vi "Set Height.vi"(8 "Error In":errorcluster, 10 "Height":u32, 11 "Square In":refnum<class "Square.lvclass">) -> (0 "Error Out":errorcluster, 3 "Square Out":refnum<class "Square.lvclass">)   [LabVIEW 2019, in "Square.lvclass"]
uses:
  Square.lvclass
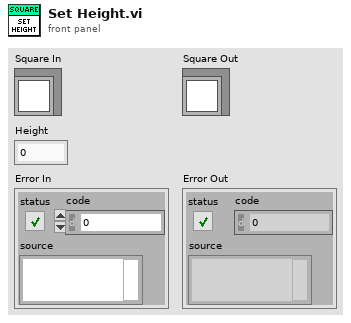
[diagram p1: front panel]
types:
  T1 = typedef "Square.lvclass/Data.ctl" = cluster{"Height":u32, "Width":u32}
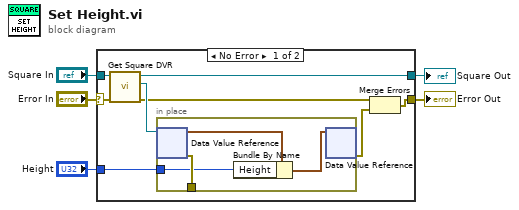
[diagram p0: block diagram]
diagram:
  n1 = case shown="No Error" "Error In" {
    selector: "Error In" -> [w9 w18]
    tunnel: [w12 w18] -> w4
    tunnel: [w7 w19] -> w2
    tunnel: "Square In" -> [w10 w19]
    tunnel: "Height" -> [w11 _]
    frame No Error {
      n2 = call "Get Square DVR.vi"("Error In"=w9, "Square In"=w10) -> ("Error Out"=w6:errorcluster, "DVR"=w8:refnum<data-value>, "Square Out"=w7:refnum<class "Square.lvclass">)  [unwired: 7 in]
      n3 = in-place {
        in-place-border: [w17] -> _
        in-place-border: w11 -> [w14]
        n4 = in-place-dvr #1(w8) -> (w16:T1, w17:errorcluster)
        n5 = Bundle By Name(cluster=w16, "Height"=w14) -> (w15:T1)
        n6 = in-place-dvr #1(w15) -> (w13:errorcluster)  [unwired: 1 out]
      }
      n7 = Merge Errors(w6, w13) -> (w12:errorcluster)
    }
    frame Error {
    }
  }
  "Square Out" <- w2
  "Error Out" <- w4
